vi "stringadd.vi"(4 "Report Data.Degree":dbl[][](array[numeric]), 5 "Mode":bool, 6 "s/d setting":bool, 7 "Str Refnum":refnum<vi>, 9 "variant":variant, 10 "Numeric":i32, 11 "String":string) -> ()   [LabVIEW 2015]
uses:
  Typedef/Inst. Queue.ctl
panel:
  in  "xy dynamic array":T1(array[cluster])
  in  "output cluster 2":cluster{T2, T2}
  out "resulting string":string
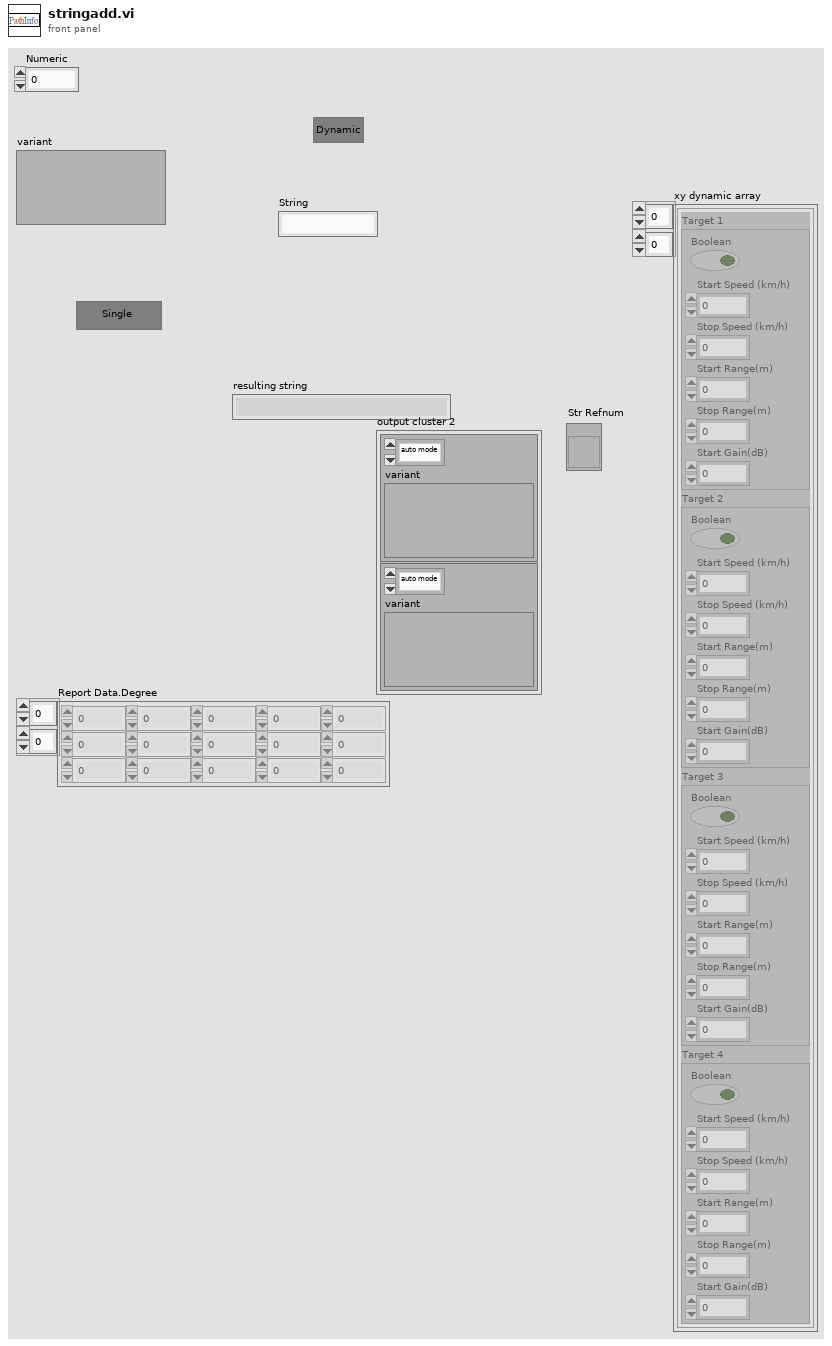
[diagram p1: front panel]
types:
  T1 = cluster{"Target 1":cluster{"Boolean":bool, "Start Speed (km/h)":dbl, "Stop Speed (km/h)":dbl, "Start Range(m)":dbl, "Stop Range(m)":dbl, "Start Gain(dB)":dbl}, "Target 2":cluster{"Boolean":bool, "Start Speed (km/h)":dbl, "Stop Speed (km/h)":dbl, "Start Range(m)":dbl, "Stop Range(m)":dbl, "Start Gain(dB)":dbl}, "Target 3":cluster{"Boolean":bool, "Start Speed (km/h)":dbl, "Stop Speed (km/h)":dbl, "Start Range(m)":dbl, "Stop Range(m)":dbl, "Start Gain(dB)":dbl}, "Target 4":cluster{"Boolean":bool, "Start Speed (km/h)":dbl, "Stop Speed (km/h)":dbl, "Start Range(m)":dbl, "Stop Range(m)":dbl, "Start Gain(dB)":dbl}}[][]
  T2 = typedef "Inst. Queue.ctl" = cluster{enum16{"auto mode", "Idle", "Inst. Connect", "£m Data", "Inst. Update", "Freq. (GHz)", "rx att", "GTX (dB)", "GRX (dB)", "Range Trim(m)", "Gain Trim (dB)", "Distance to RUT", "Mapping", "Convert", "RF ON/OFF", "Run", "Direct Program", "Stop", "Dynamic", "dyset", "Exit"}, "variant":variant}
  T3 = cluster{"target D_1":cluster{"Boolean":bool, "Start Speed (km/h)":dbl, "Stop Speed (km/h)":dbl, "Start Range(m)":dbl, "Stop Range(m)":dbl, "Start Gain(dB)":dbl}, "target D_2":cluster{"Boolean":bool, "Start Speed (km/h)":dbl, "Stop Speed (km/h)":dbl, "Start Range(m)":dbl, "Stop Range(m)":dbl, "Start Gain(dB)":dbl}, "target D_3":cluster{"Boolean":bool, "Start Speed (km/h)":dbl, "Stop Speed (km/h)":dbl, "Start Range(m)":dbl, "Stop Range(m)":dbl, "Start Gain(dB)":dbl}, "target D_4":cluster{"Boolean":bool, "Start Speed (km/h)":dbl, "Stop Speed (km/h)":dbl, "Start Range(m)":dbl, "Stop Range(m)":dbl, "Start Gain(dB)":dbl}}
  T4 = cluster{"Target 1":cluster{"Boolean":bool, "Speed":dbl, "Range":dbl, "Gain":dbl}, "Target 2":cluster{"Boolean":bool, "Speed":dbl, "Range":dbl, "Gain":dbl}, "Target 3":cluster{"Boolean":bool, "Speed":dbl, "Range":dbl, "Gain":dbl}, "Target 4":cluster{"Boolean":bool, "Speed":dbl, "Range":dbl, "Gain":dbl}}
  T5 = cluster{"Boolean":bool, "Start Speed (km/h)":dbl, "Stop Speed (km/h)":dbl, "Start Range(m)":dbl, "Stop Range(m)":dbl, "Start Gain(dB)":dbl}
  T6 = cluster{"Boolean":bool, "Speed":dbl, "Range":dbl, "Gain":dbl}
  T7 = cluster{"Target 1":cluster{"Boolean":bool, "Start Speed (km/h)":dbl, "Stop Speed (km/h)":dbl, "Start Range(m)":dbl, "Stop Range(m)":dbl, "Start Gain(dB)":dbl}, "Target 2":cluster{"Boolean":bool, "Start Speed (km/h)":dbl, "Stop Speed (km/h)":dbl, "Start Range(m)":dbl, "Stop Range(m)":dbl, "Start Gain(dB)":dbl}, "Target 3":cluster{"Boolean":bool, "Start Speed (km/h)":dbl, "Stop Speed (km/h)":dbl, "Start Range(m)":dbl, "Stop Range(m)":dbl, "Start Gain(dB)":dbl}, "Target 4":cluster{"Boolean":bool, "Start Speed (km/h)":dbl, "Stop Speed (km/h)":dbl, "Start Range(m)":dbl, "Stop Range(m)":dbl, "Start Gain(dB)":dbl}}[]
  T8 = cluster{"Target 1":cluster{"Boolean":bool, "Start Speed (km/h)":dbl, "Stop Speed (km/h)":dbl, "Start Range(m)":dbl, "Stop Range(m)":dbl, "Start Gain(dB)":dbl}, "Target 2":cluster{"Boolean":bool, "Start Speed (km/h)":dbl, "Stop Speed (km/h)":dbl, "Start Range(m)":dbl, "Stop Range(m)":dbl, "Start Gain(dB)":dbl}, "Target 3":cluster{"Boolean":bool, "Start Speed (km/h)":dbl, "Stop Speed (km/h)":dbl, "Start Range(m)":dbl, "Stop Range(m)":dbl, "Start Gain(dB)":dbl}, "Target 4":cluster{"Boolean":bool, "Start Speed (km/h)":dbl, "Stop Speed (km/h)":dbl, "Start Range(m)":dbl, "Stop Range(m)":dbl, "Start Gain(dB)":dbl}}
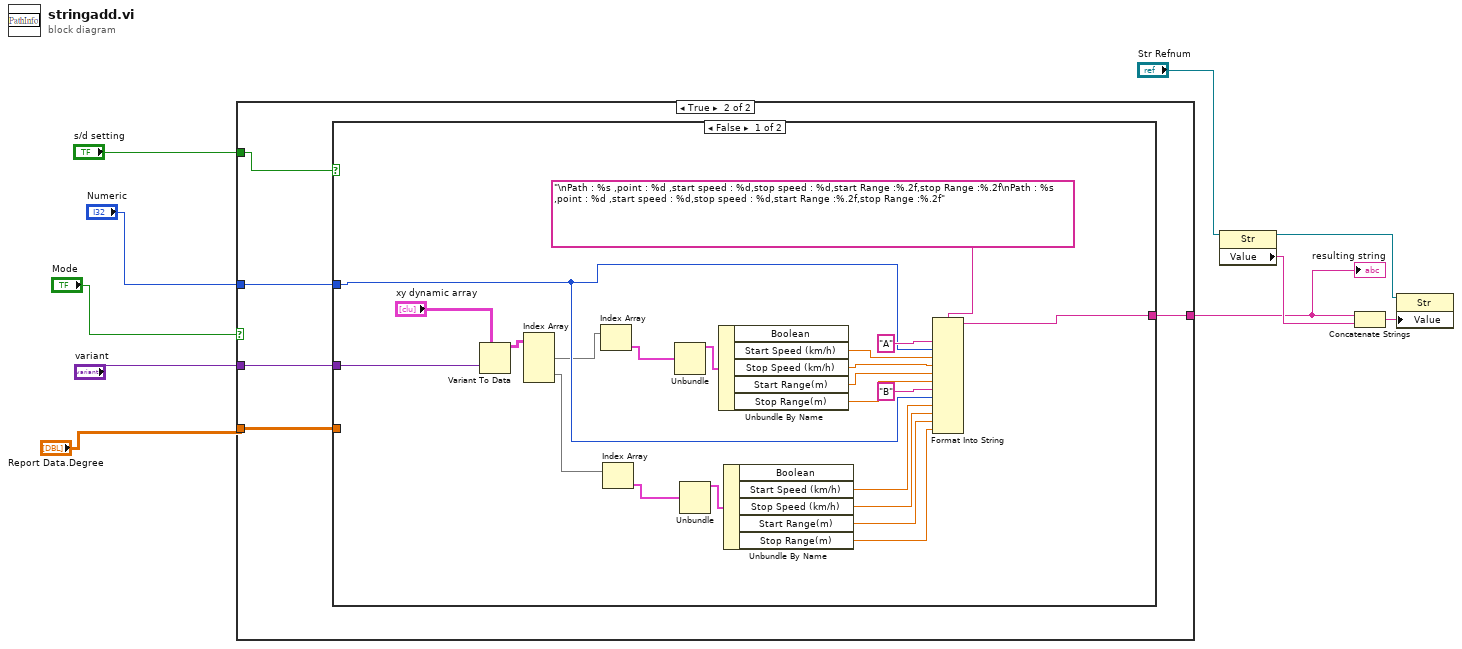
[diagram p0: block diagram]
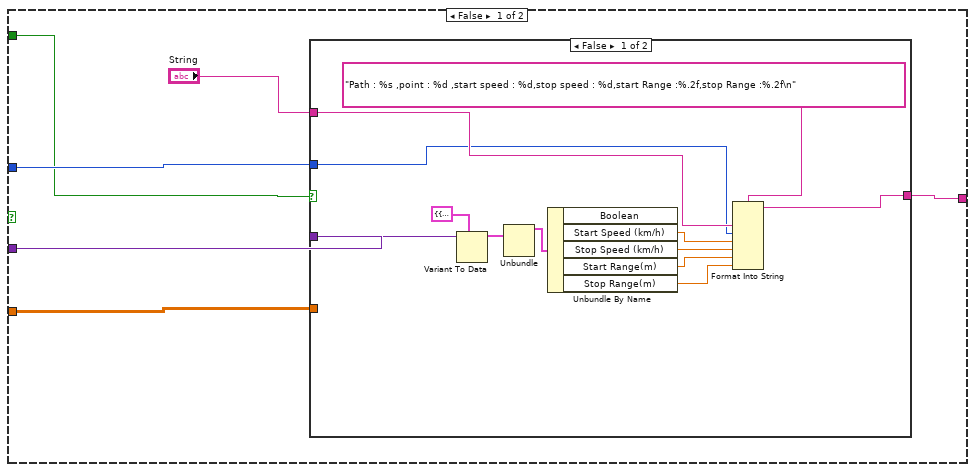
[diagram p2: hidden frame]
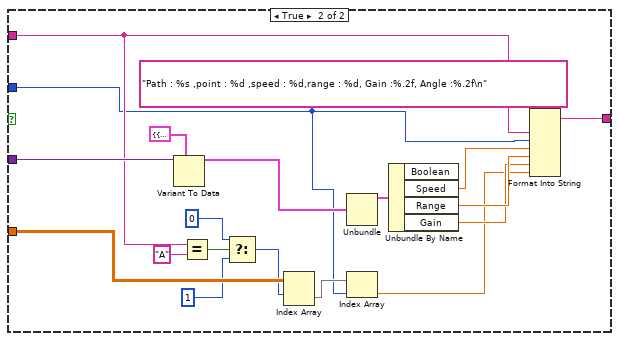
[diagram p3: hidden frame]
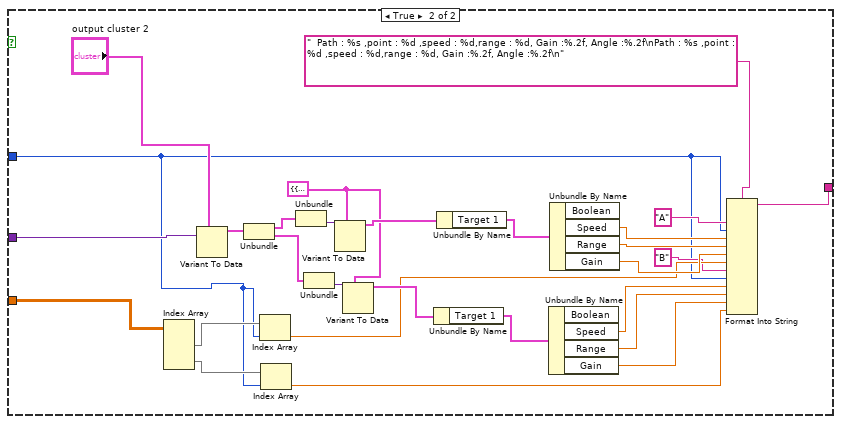
[diagram p4: hidden frame]
diagram:
  n1 = case shown="True" "Mode" {
    tunnel: [w16 w52] -> w7
    tunnel: "variant" -> [w14 w51]
    tunnel: "Numeric" -> [w13 w49]
    tunnel: "Report Data.Degree" -> [w12 w50]
    tunnel: "s/d setting" -> [w11 w48]
    frame False {
      n2 = case shown="False" w11 {
        tunnel: w14 -> [w28 w41]
        tunnel: [w18 w39] -> w16
        tunnel: "String" -> [w23 w37]
        tunnel: w13 -> [w22 w29]
        tunnel: w12 -> [_ w35]
        frame False {
          n3 = Variant To Data(type=T3 {"target D_1"={"Boolean"=FALSE, "Start Speed (km/h)"=0.0, "Stop Speed (km/h)"=0.0, "Start Range(m)"=0.0, "Stop Range(m)"=0.0, "Start Gain(dB)"=0.0}, "target D_2"={"Boolean"=FALSE, "Start Speed (km/h)"=0.0, "Stop Speed (km/h)"=0.0, "Start Range(m)"=0.0, "Stop Range(m)"=0.0, "Start Gain(dB)"=0.0}, "target D_3"={"Boolean"=FALSE, "Start Speed (km/h)"=0.0, "Stop Speed (km/h)"=0.0, "Start Range(m)"=0.0, "Stop Range(m)"=0.0, "Start Gain(dB)"=0.0}, "target D_4"={"Boolean"=FALSE, "Start Speed (km/h)"=0.0, "Stop Speed (km/h)"=0.0, "Start Range(m)"=0.0, "Stop Range(m)"=0.0, "Start Gain(dB)"=0.0}} ("dynamic  2"), Variant=w28) -> (data=w25:T3)  [unwired: 1 in, 1 out]
          n4 = Unbundle(w25) -> ("target D_1"=w24:T5)  [unwired: 3 out]
          n5 = Unbundle By Name(w24) -> ("Start Speed (km/h)"=w21:dbl, "Stop Speed (km/h)"=w20:dbl, "Start Range(m)"=w19:dbl, "Stop Range(m)"=w17:dbl)  [unwired: 1 out]
          n6 = Format Into String(format string="Path : %s ,point : %d ,start speed : %d,stop speed : %d,start Range :%.2f,stop Range :%.2f\n", w23, w22, w21, w20, w19, w17) -> (resulting string=w18:string)  [unwired: 2 in, 1 out]
        }
        frame True {
          n7 = Variant To Data(type=T4 {"Target 1"={"Boolean"=TRUE, "Speed"=0.0, "Range"=0.0, "Gain"=0.0}, "Target 2"={"Boolean"=TRUE, "Speed"=0.0, "Range"=0.0, "Gain"=0.0}, "Target 3"={"Boolean"=TRUE, "Speed"=0.0, "Range"=0.0, "Gain"=0.0}, "Target 4"={"Boolean"=TRUE, "Speed"=0.0, "Range"=0.0, "Gain"=0.0}} ("Direct program 2"), Variant=w41) -> (data=w40:T4)  [unwired: 1 in, 1 out]
          n8 = Equal?(x=w37, y="A") -> (x = y?=w38:bool)
          n9 = Select(t=0, s=w38, f=1) -> (s? t:f=w32:i32)
          n10 = Index Array(array=w35, index (row)=w32) -> (element=w31:dbl[])  [unwired: 1 in]
          n11 = Unbundle(w40) -> ("Target 1"=w47:T6)  [unwired: 3 out]
          n12 = Index Array(array=w31, index=w29) -> (element=w30:dbl)
          n13 = Unbundle By Name(w47) -> ("Speed"=w45:dbl, "Range"=w44:dbl, "Gain"=w43:dbl)  [unwired: 1 out]
          n14 = Format Into String(format string="Path : %s ,point : %d ,speed : %d,range : %d, Gain :%.2f, Angle :%.2f\n", w37, w29, w45, w44, w43, w30) -> (resulting string=w39:string)  [unwired: 2 in, 1 out]
        }
      }
    }
    frame True {
      n15 = case shown="False" w48 {
        tunnel: [w64 w102] -> w52
        tunnel: w51 -> [w72 w101]
        tunnel: w50 -> [_ w81]
        tunnel: w49 -> [w69 w75]
        frame False {
          n16 = Variant To Data(type="xy dynamic array", Variant=w72) -> (data=w62:T1)  [unwired: 1 in, 1 out]
          n17 = Index Array(array=w62) -> (element #1=w61:T7, element #2=w59:T7)  [unwired: 4 in]
          n18 = Index Array(array=w61) -> (element=w60:T8)  [unwired: 1 in]
          n19 = Index Array(array=w59) -> (element=w57:T8)  [unwired: 1 in]
          n20 = Unbundle(w60) -> ("Target 1"=w73:T5)  [unwired: 3 out]
          n21 = Unbundle(w57) -> ("Target 1"=w58:T5)  [unwired: 3 out]
          n22 = Unbundle By Name(w73) -> ("Start Speed (km/h)"=w68:dbl, "Stop Speed (km/h)"=w67:dbl, "Start Range(m)"=w66:dbl, "Stop Range(m)"=w65:dbl)  [unwired: 1 out]
          n23 = Unbundle By Name(w58) -> ("Start Speed (km/h)"=w56:dbl, "Stop Speed (km/h)"=w55:dbl, "Start Range(m)"=w54:dbl, "Stop Range(m)"=w53:dbl)  [unwired: 1 out]
          n24 = Format Into String(format string="\nPath : %s ,point : %d ,start speed : %d,stop speed : %d,start Range :%.2f,stop Range :%.2f\nPath : %s ,point : %d ,start speed : %d,stop speed : %d,start Range :%.2f,stop Range :%.2f", "A" ("input 1"), w69, w68, w67, w66, w65, "B" ("input 7"), w69, w56, w55, w54, w53) -> (resulting string=w64:string)  [unwired: 2 in, 1 out]
        }
        frame True {
          w87 = T4 {"Target 1"={"Boolean"=TRUE, "Speed"=0.0, "Range"=0.0, "Gain"=0.0}, "Target 2"={"Boolean"=TRUE, "Speed"=0.0, "Range"=0.0, "Gain"=0.0}, "Target 3"={"Boolean"=TRUE, "Speed"=0.0, "Range"=0.0, "Gain"=0.0}, "Target 4"={"Boolean"=TRUE, "Speed"=0.0, "Range"=0.0, "Gain"=0.0}} ("Direct program 2")
          n25 = Index Array(array=w81) -> (element #1=w80:dbl[], element #2=w79:dbl[])  [unwired: 4 in]
          n26 = Variant To Data(type="output cluster 2", Variant=w101) -> (data=w94:cluster{T2, T2})  [unwired: 1 in, 1 out]
          n27 = Unbundle(w94) -> (w92:T2, w89:T2)
          n28 = Index Array(array=w80, index=w75) -> (element=w78:dbl)
          n29 = Index Array(array=w79, index=w75) -> (element=w77:dbl)
          n30 = Unbundle(w92) -> ("variant"=w91:variant)  [unwired: 1 out]
          n31 = Unbundle(w89) -> ("variant"=w90:variant)  [unwired: 1 out]
          n32 = Variant To Data(type=w87, Variant=w91) -> (data=w88:T4)  [unwired: 1 in, 1 out]
          n33 = Variant To Data(type=w87, Variant=w90) -> (data=w86:T4)  [unwired: 1 in, 1 out]
          n34 = Unbundle By Name(w86) -> ("Target 1"=w95:T6)
          n35 = Unbundle By Name(w88) -> ("Target 1"=w99:T6)
          n36 = Unbundle By Name(w95) -> ("Speed"=w84:dbl, "Range"=w83:dbl, "Gain"=w82:dbl)  [unwired: 1 out]
          n37 = Unbundle By Name(w99) -> ("Speed"=w98:dbl, "Range"=w97:dbl, "Gain"=w85:dbl)  [unwired: 1 out]
          n38 = Format Into String(format string="  Path : %s ,point : %d ,speed : %d,range : %d, Gain :%.2f, Angle :%.2f\nPath : %s ,point : %d ,speed : %d,range : %d, Gain :%.2f, Angle :%.2f\n", "A" ("input 1"), w75, w98, w97, w85, w78, "B" ("input 6"), w75, w84, w83, w82, w77) -> (resulting string=w102:string)  [unwired: 2 in, 1 out]
        }
      }
    }
  }
  "resulting string" <- w7
  n39 = property class="Str"(reference="Str Refnum") -> (reference out=w6:refnum<vi>, "Value"=w8:string)  [unwired: 1 in, 1 out]
  n40 = Concatenate Strings(w7, w8) -> (w10:string)
  n41 = property class="Str"(reference=w6, "Value"=w10) -> ()  [unwired: 1 in, 2 out]
